vi "Teleop.vi"(10 "Match Info":T1={"Autonomous Elapsed Seconds"=0.0, "TeleOp Elapsed Seconds"=0.0, "Disabled Elapsed Seconds"=0.0, "Visited Autonomous"=FALSE, "Visited TeleOp"=FALSE, "Visited Disabled"=FALSE, "Autonomous Settings"={"Autonomous Style"=enum."Independent", "VI Refnum"=refnum}}, 11 "Call Context":T2) -> ()   [LabVIEW 2012]
doc: "This VI is called for each TeleOp packet received from the DS where the robot is not disabled. It is often used to read from the joysticks and update I/O or to update setpoints for timed control loops. It should complete and return within 20 milliseconds or it may miss DS packets."
uses:
  <vilib>/Rock Robotics/WPI/DriverStation/WPI_DriverStationDerivedRobotMode.ctl
  <vilib>/Rock Robotics/WPI/DriverStation/WPI_DriverStationMatch Info.ctl
  <vilib>/Rock Robotics/SystemInterfaces/Utilities/FPGA_UtilitiesLED Source.ctl
  Robot Global Data.vi
  <vilib>/Rock Robotics/WPI/Joystick/WPI_JoystickGetSetRefNum.vi
  <vilib>/Rock Robotics/WPI/RobotDrive/WPI_RobotDriveGetSetRefNum.vi
panel:
  in  "Current X Motor Speed (-1 to 1)":dbl
  in  "Current Y Motor Speed (-1 to 1)":dbl
  out "Numeric 1":dbl(slide) scale=0.0..100.0
  out "Boolean 2":bool
  out "Boolean 1":bool
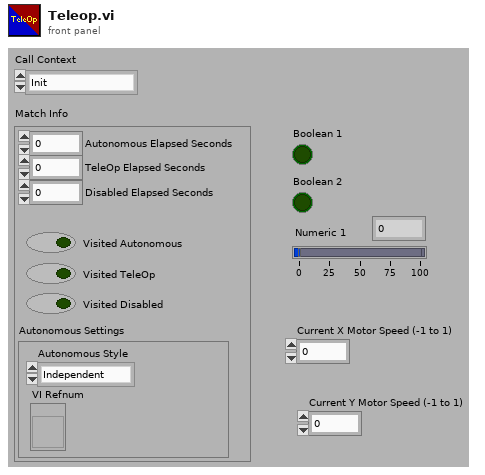
[diagram p1: front panel]
types:
  T1 = typedef "WPI_DriverStationMatch Info.ctl" = cluster{"Autonomous Elapsed Seconds":dbl, "TeleOp Elapsed Seconds":dbl, "Disabled Elapsed Seconds":dbl, "Visited Autonomous":bool, "Visited TeleOp":bool, "Visited Disabled":bool, "Autonomous Settings":cluster{"Autonomous Style":enum16{"Iterative", "Independent"}, "VI Refnum":refnum<vi>}}
  T2 = typedef "WPI_DriverStationDerivedRobotMode.ctl" = enum16{"Init", "Execute", "Stop"}
  T3 = typedef "FPGA_UtilitiesLED Source.ctl" = enum16{"User LED", "FPGA LED"}
  T4 = typedef "WPI_JoystickDevRef.ctl" = cluster{"Device":T5}
  T5 = typedef "WPI_JoystickDeviceEnum.ctl" = enum16{"USB 1", "USB 2", "USB 3", "USB 4", "Kinect 1", "Kinect 2"}
  T6 = typedef "WPI_JoystickButtonState.ctl" = cluster{"Button 1":bool, "Button 2":bool, "Button 3":bool, "Button 4":bool, "Button 5":bool, "Button 6":bool, "Button 7":bool, "Button 8":bool, "Button 9":bool, "Button 10":bool, "Button 11":bool, "Button 12":bool}
  T7 = typedef "WPI_MotorControlDeviceRef.ctl" = cluster{"DeviceStatus":errorcluster, "Type":enum16{"PWM", "CAN"}, "PWM":cluster{"Digital Module":T8, "PWM Channel":T9, "DeadBand":T10}, "CAN":cluster{"Device Number":u8, "Control Mode":T11, "Semaphore":T12, "Max Vout":dbl}, "Invert":bool, "TransformRef":T13, "InvTransformRef":T13}
  T8 = typedef "FPGA_TypedefDigitalModule.ctl" = enum16{"Digital Module 1", "Digital Module 2"}
  T9 = typedef "FPGA_DIOPWMChannel.ctl" = enum8{"PWM 1", "PWM 2", "PWM 3", "PWM 4", "PWM 5", "PWM 6", "PWM 7", "PWM 8", "PWM 9", "PWM 10", "Invalid"}
  T10 = typedef "WPI_PWMDeadband.ctl" = cluster{"Name":string, "maxPositivePwm":i32, "minPositivePwm":i32, "centerPwm":i32, "maxNegativePwm":i32, "minNegativePwm":i32, "angularRange":u16}
  T11 = typedef "WPI_CANJaguar_ControlMode.ctl" = enum8{"Percent VBus", "Current", "Speed", "Position", "Voltage"}
  T12 = typedef "Semaphore RefNum" = refnum<k1>
  T13 = typedef "WPI_PWMTransform_ConPane.ctl" = refnum<vi>
  T14 = typedef "WPI_RobotDriveDevRef.ctl" = cluster{"DevStatus":errorcluster, "Motors[]":T7[], "Square Inputs":bool, "Max Output":dbl, "Isochronous":bool}
  T15 = cluster{"axis 1 (x)":dbl, "axis 2 (y)":dbl, "axis 3 (throttle)":dbl, "axis 4":dbl, "axis 5":dbl, "axis 6":dbl}
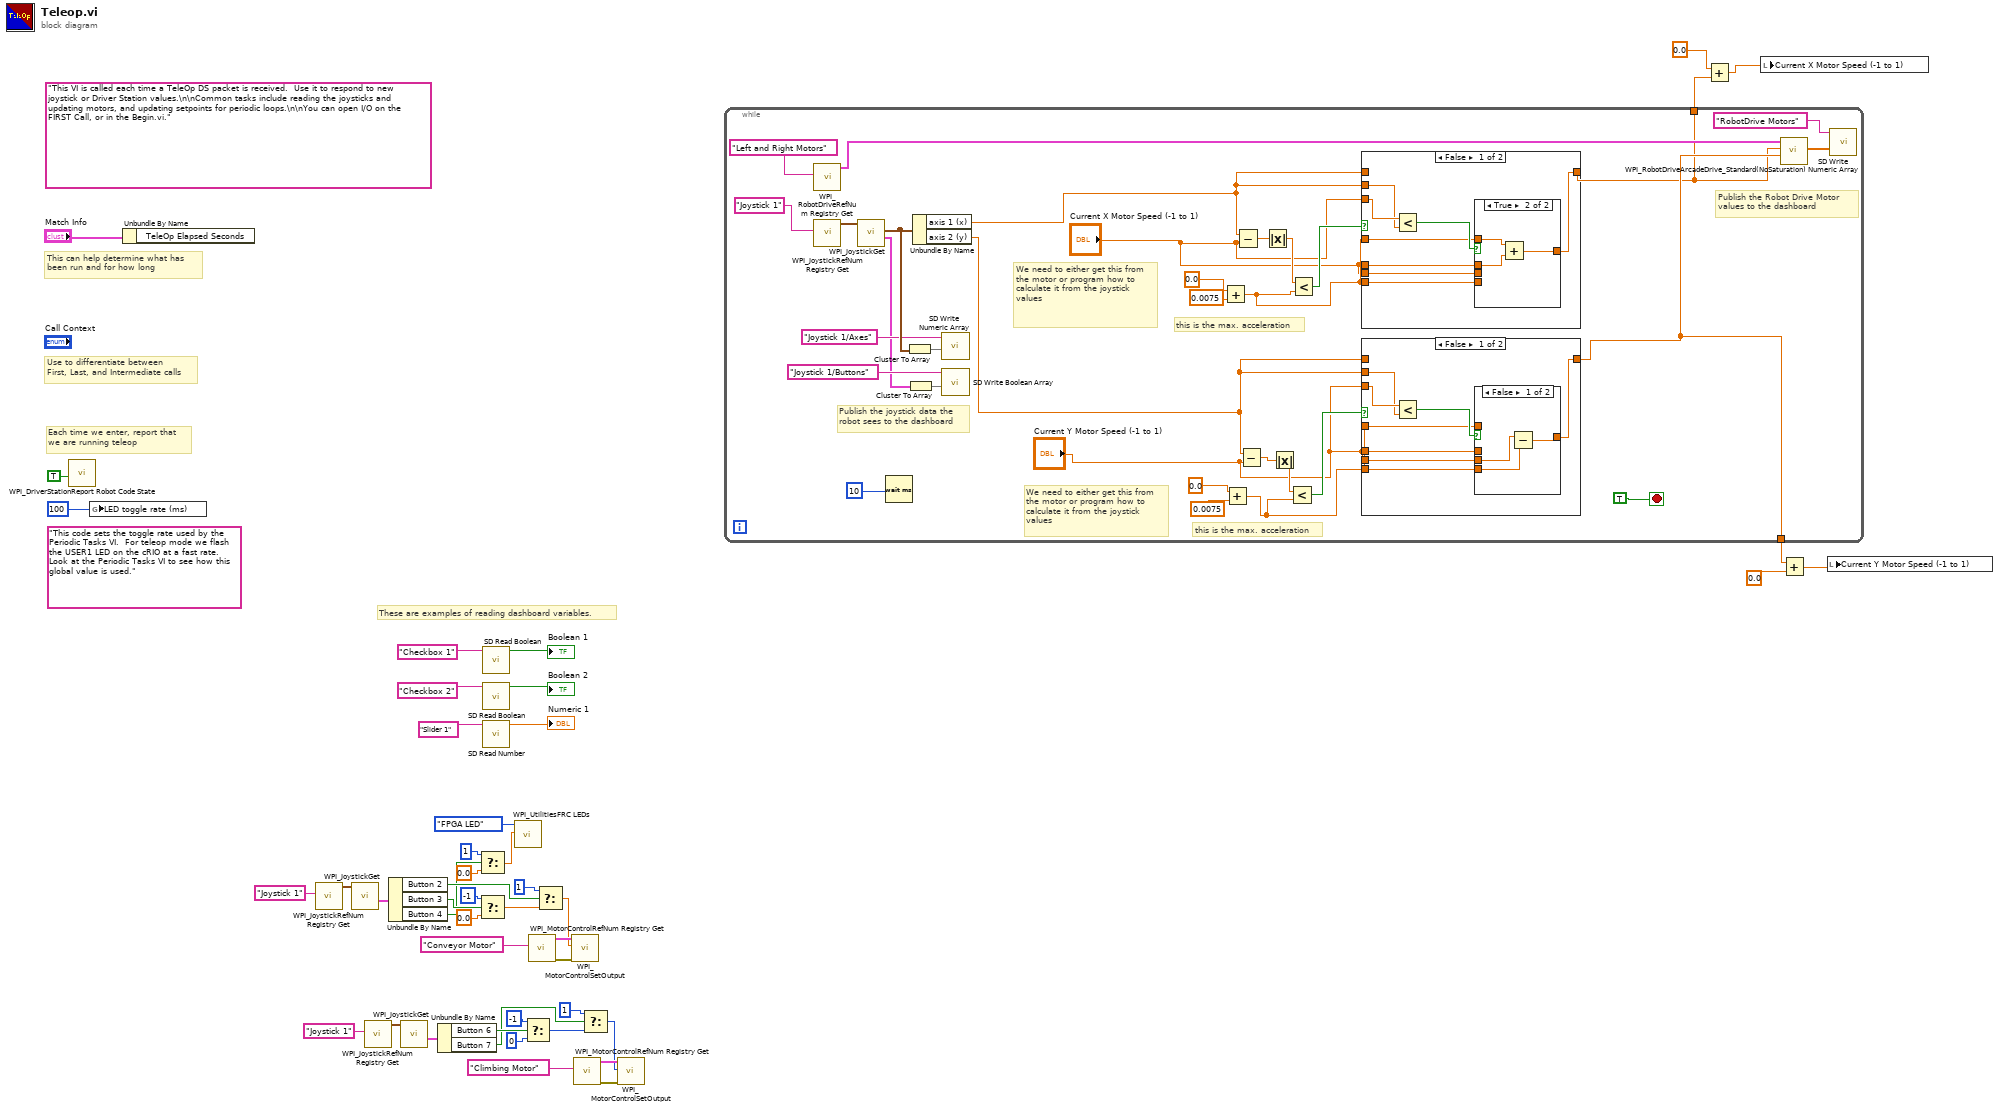
[diagram p0: block diagram]
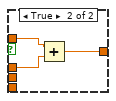
[diagram p2: hidden frame]
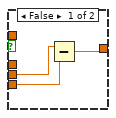
[diagram p4: hidden frame]
diagram:
  (unwired) "This code sets the toggle rate used by the Periodic Tasks VI.  For teleop mode we flash the USER1 LED on the cRIO at a fast rate.  Look at the Periodic Tasks VI to see how this global value is used."
  (unwired) "This VI is called each time a TeleOp DS packet is received.  Use it to respond to new joystick or Driver Station values.\n\nCommon tasks include reading the joysticks and updating motors, and updating setpoints for periodic loops.\n\nYou can open I/O on the FIRST Call, or in the Begin.vi."
  # "These are examples of reading dashboard variables."
  # "Each time we enter, report that\nwe are running teleop"
  # "Use to differentiate between\nFirst, Last, and Intermediate calls"
  # "This can help determine what has\nbeen run and for how long"
  n1 = call <vilib>:"WPI_DriverStationReport Robot Code State.vi"("TeleOp"=TRUE ("Autonomous")) -> ()  [unwired: 10 in, 1 out]
  n2 = global write "Robot Global Data.vi" "LED toggle rate (ms)"(u32 100 ("LED ms toggle rate")) -> ()
  n3 = Unbundle By Name("Match Info") -> ()  [unwired: 1 out]
  n4 = call <vilib>:"WPI_JoystickRefNum Registry Get.vi"("refnum name"="Joystick 1") -> ("JoystickDevRef"=w37:T4)  [unwired: 9 in, 1 out]
  n5 = call <vilib>:"WPI_JoystickGet.vi"("JoystickDevRef"=w37) -> ("Buttons"=w36:T6)  [unwired: 4 in, 2 out]
  n6 = call <vilib>:"WPI_JoystickRefNum Registry Get.vi"("refnum name"="Joystick 1") -> ("JoystickDevRef"=w18:T4)  [unwired: 9 in, 1 out]
  n7 = Unbundle By Name(w36) -> ("Button 2"=w35:bool, "Button 3"=w32:bool, "Button 4"=w23:bool)
  n8 = call <vilib>:"WPI_JoystickGet.vi"("JoystickDevRef"=w18) -> ("Buttons"=w17:T6)  [unwired: 4 in, 2 out]
  n9 = Unbundle By Name(w17) -> ("Button 6"=w16:bool, "Button 7"=w15:bool)
  n10 = Select(t=1, s=w23, f=0.0) -> (s? t:f=w22:dbl)
  n11 = Select(t=-1, s=w32, f=0.0) -> (s? t:f=w30:dbl)
  n12 = call <vilib>:"SD Read Boolean.vi"("Name"="Checkbox 1" ("refnum name")) -> ("Boolean"=→"Boolean 1":bool)  [unwired: 8 in, 2 out]
  n13 = call <vilib>:"SD Read Boolean.vi"("Name"="Checkbox 2" ("refnum name")) -> ("Boolean"=→"Boolean 2":bool)  [unwired: 8 in, 2 out]
  n14 = call <vilib>:"SD Read Number.vi"("Name"="Slider 1" ("refnum name")) -> ("Numeric"=→"Numeric 1":dbl)  [unwired: 8 in, 2 out]
  n15 = call <vilib>:"WPI_UtilitiesFRC LEDs.vi"("State"=w22, "LED Type"=FPGA_UtilitiesLED_Source."FPGA LED") -> ()  [unwired: 1 in, 9 out]
  n16 = Select(t=-1, s=w16, f=0) -> (s? t:f=w10:i32)
  n17 = call <vilib>:"WPI_MotorControlRefNum Registry Get.vi"("refnum name"="Conveyor Motor") -> ("error out"=w29:errorcluster, "MotorControlDevRef"=w28:T7)  [unwired: 9 in]
  n18 = Select(t=1, s=w35, f=w30) -> (s? t:f=w27:dbl)
  n19 = call <vilib>:"WPI_MotorControlSetOutput.vi"("error in (no error)"=w29, "Output"=w27, "MotorControlDevRef"=w28) -> ()  [unwired: 6 in, 3 out]
  n20 = call <vilib>:"WPI_MotorControlRefNum Registry Get.vi"("refnum name"="Climbing Motor") -> ("error out"=w11:errorcluster, "MotorControlDevRef"=w12:T7)  [unwired: 9 in]
  n21 = Select(t=1, s=w15, f=w10) -> (s? t:f=w7:i32)
  n22 = call <vilib>:"WPI_MotorControlSetOutput.vi"("error in (no error)"=w11, "Output"=w7, "MotorControlDevRef"=w12) -> ()  [unwired: 6 in, 3 out]
  n23 = while {
    tunnel: [w48] -> w4
    tunnel: [w47] -> w2
    stop <- TRUE stop-if-true
    # "We need to either get this from the motor or program how to calculate it from the joystick values"
    # "this is the max. acceleration"
    # "We need to either get this from the motor or program how to calculate it from the joystick values"
    # "this is the max. acceleration"
    # "Publish the Robot Drive Motor\nvalues to the dashboard"
    # "Publish the joystick data the\nrobot sees to the dashboard"
    n24 = call <vilib>:"WPI_RobotDriveRefNum Registry Get.vi"("refnum name"="Left and Right Motors") -> ("RobotDriveDevRef"=w61:T14)  [unwired: 1 in, 9 out]
    n25 = call <vilib>:"WPI_JoystickRefNum Registry Get.vi"("refnum name"="Joystick 1") -> ("JoystickDevRef"=w76:T4)  [unwired: 1 in, 9 out]
    n26 = call <vilib>:"WPI_JoystickGet.vi"("JoystickDevRef"=w76) -> ("Buttons"=w68:T6, "Axes"=w73:T15)  [unwired: 1 in, 4 out]
    n27 = Wait (ms)(milliseconds to wait=10) -> ()  [unwired: 1 out]
    n28 = Cluster To Array(cluster=w73) -> (array=w72:dbl[])
    n29 = Cluster To Array(cluster=w68) -> (array=w75:bool[])
    n30 = Unbundle By Name(w73) -> ("axis 1 (x)"=w62:dbl, "axis 2 (y)"=w57:dbl)
    n31 = call <vilib>:"SD Write Numeric Array.vi"("Numeric Array"=w72, "Name"="Joystick 1/Axes") -> ()  [unwired: 8 in, 2 out]
    n32 = call <vilib>:"SD Write Boolean Array.vi"("Boolean Array"=w75, "Name"="Joystick 1/Buttons") -> ()  [unwired: 8 in, 2 out]
    n33 = Add(x=0.0, y=0.0075) -> (x+y=w54:dbl)
    n34 = Add(x=0.0, y=0.0075) -> (x+y=w51:dbl)
    n35 = Subtract(x=w62, y="Current X Motor Speed (-1 to 1)") -> (x-y=w55:dbl)
    n36 = Subtract(x=w57, y="Current Y Motor Speed (-1 to 1)") -> (x-y=w52:dbl)
    n37 = Absolute Value(x=w55) -> (abs(x)=w56:dbl)
    n38 = Absolute Value(x=w52) -> (abs(x)=w53:dbl)
    n39 = Less?(x=w53, y=w51) -> (x < y?=w58:bool)
    n40 = Less?(x=w56, y=w54) -> (x < y?=w63:bool)
    n41 = case shown="False" w63 {
      tunnel: [w96 w108] -> w47
      tunnel: w62 -> [_ w108]
      tunnel: "Current X Motor Speed (-1 to 1)" -> [w101 _]
      tunnel: w62 -> [w100 _]
      tunnel: "Current X Motor Speed (-1 to 1)" -> [w98 _]
      tunnel: w54 -> [w97 _]
      tunnel: "Current X Motor Speed (-1 to 1)" -> [w95 _]
      tunnel: w54 -> [w94 _]
      frame False {
        n42 = Less?(x=w101, y=w100) -> (x < y?=w99:bool)
        n43 = case shown="True" w99 {
          tunnel: w98 -> [_ w107]
          tunnel: w97 -> [_ w106]
          tunnel: [w104 w105] -> w96
          tunnel: w95 -> [w103 _]
          tunnel: w94 -> [w102 _]
          frame False {
            n44 = Subtract(x=w103, y=w102) -> (x-y=w104:dbl)
          }
          frame True {
            n45 = Add(x=w106, y=w107) -> (x+y=w105:dbl)
          }
        }
      }
      frame True {
      }
    }
    n46 = case shown="False" w58 {
      tunnel: [w81 w93] -> w48
      tunnel: w57 -> [_ w93]
      tunnel: "Current Y Motor Speed (-1 to 1)" -> [w86 _]
      tunnel: w57 -> [w85 _]
      tunnel: "Current Y Motor Speed (-1 to 1)" -> [w83 _]
      tunnel: w51 -> [w82 _]
      tunnel: "Current Y Motor Speed (-1 to 1)" -> [w80 _]
      tunnel: w51 -> [w79 _]
      frame False {
        n47 = Less?(x=w86, y=w85) -> (x < y?=w84:bool)
        n48 = case shown="False" w84 {
          tunnel: w83 -> [_ w92]
          tunnel: w82 -> [_ w91]
          tunnel: [w89 w90] -> w81
          tunnel: w80 -> [w88 _]
          tunnel: w79 -> [w87 _]
          frame False {
            n49 = Subtract(x=w88, y=w87) -> (x-y=w89:dbl)
          }
          frame True {
            n50 = Add(x=w91, y=w92) -> (x+y=w90:dbl)
          }
        }
      }
      frame True {
      }
    }
    n51 = call <vilib>:"WPI_RobotDriveArcadeDrive_Standard(NoSaturation).vi"("Y axis value"=w48, "X axis value"=w47, "RobotDriveDevRef"=w61) -> ("Motor Values"=w69:dbl[])  [unwired: 1 in, 7 out]
    n52 = call <vilib>:"SD Write Numeric Array.vi"("Numeric Array"=w69, "Name"="RobotDrive Motors") -> ()  [unwired: 8 in, 2 out]
  }
  n53 = Add(x=0.0, y=w2) -> (x+y=w1:dbl)
  n54 = local write "Current X Motor Speed (-1 to 1)"(w1) -> ()
  n55 = Add(x=w4, y=0.0) -> (x+y=w5:dbl)
  n56 = local write "Current Y Motor Speed (-1 to 1)"(w5) -> ()
